vi "TSV_2_LV.vi"(8 "error in (no error)":errorcluster, 11 "tsv file path (dialog if empty)":path) -> (0 "error out":errorcluster, 2 "data":T2[](array[typedef]))   [LabVIEW 2019, in "VCL_2_DSC.lvclass"]
uses:
  VCL_2_DSC.lvclass
  typedefs/TSLtoLV-cluster.ctl
  <vilib>/Utility/file.llb/Read Delimited Spreadsheet (string).vi
  <userlib>/_OpenG.lib/array/array.llb/Index 1D Array Elements (String)__ogtk.vi
  <userlib>/_OpenG.lib/array/array.llb/Remove Duplicates from 1D Array (I32)__ogtk.vi
  <vilib>/Utility/file.llb/Read Delimited Spreadsheet (DBL).vi
  <userlib>/_OpenG.lib/array/array.llb/Delete Elements from 1D Array (DBL)__ogtk.vi
  <userlib>/_OpenG.lib/array/array.llb/Remove Duplicates from 1D Array (DBL)__ogtk.vi
  <userlib>/_OpenG.lib/array/array.llb/Index 1D Array Elements (Variant)__ogtk.vi
  <userlib>/_OpenG.lib/array/array.llb/Delete Elements from 1D Array (Variant)__ogtk.vi
  <userlib>/_OpenG.lib/array/array.llb/Filter 1D Array (DBL)__ogtk.vi
  <vilib>/addons/WireFlow/_WF_ProgressBar.llb/ProgressBar_WireFlow.lvclass
panel:
  in  "index 2":i32
  out "Waveform Graph":dbl[](graph)
  in  "index":i32
  out "XY Graph 2":T1(graph)
  out "XY Graph":T3(graph)
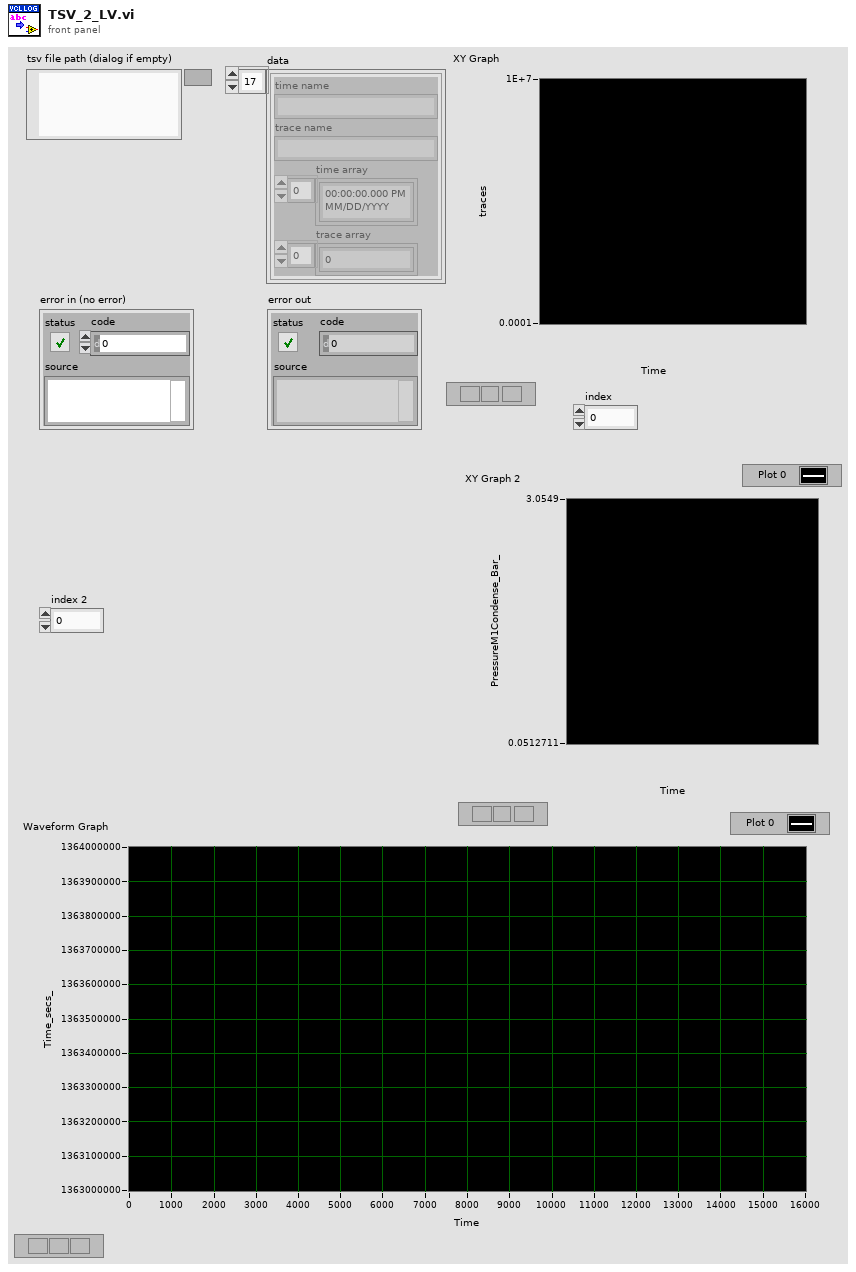
[diagram p1: front panel]
types:
  T1 = cluster{"time array":timestamp[], "trace array":dbl[]}
  T2 = typedef "VCL_2_DSC.lvclass/TSLtoLV-cluster.ctl" = cluster{"time name":string, "trace name":string, "time array":timestamp[], "trace array":dbl[]}
  T3 = cluster{"time array":timestamp[], "trace array":dbl[]}[]
  T4 = cluster{string, string, cluster{dbl[]}, cluster{dbl[]}}
  T5 = cluster{string, string, cluster{dbl[]}, cluster{dbl[]}}[]
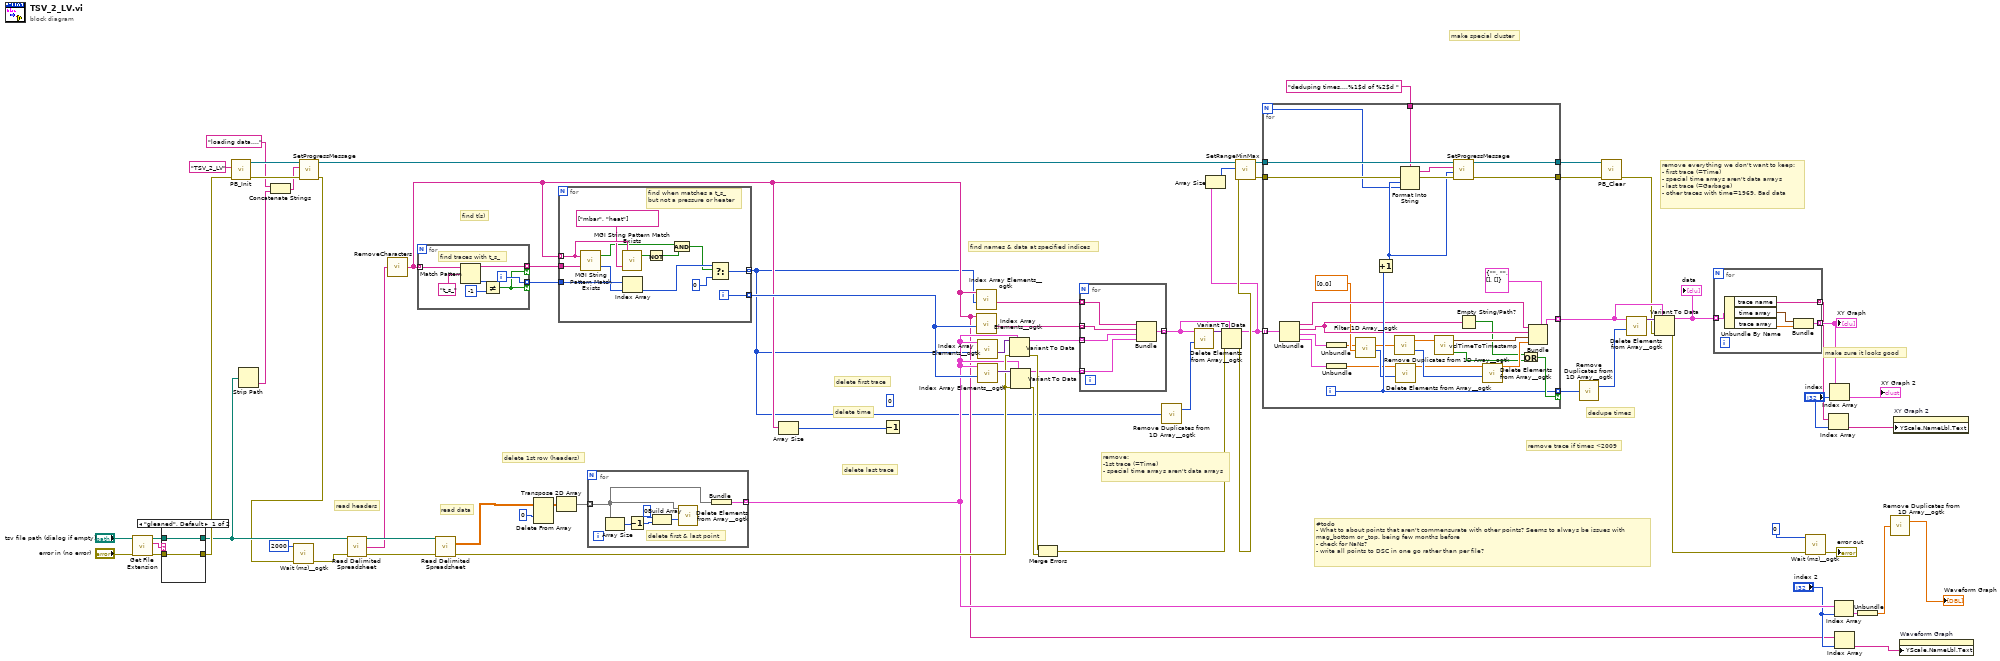
[diagram p0: block diagram]
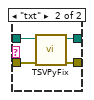
[diagram p2: hidden frame]
diagram:
  (unwired) 0 ("element")
  # "remove:\n-1st trace (=Time)\n- special time arrays aren't data arrays"
  # "#todo\n- What to about points that aren't commensurate with other points? Seems to always be issues with \nmag_bottom or _top. being few months before\n- check for NaNs?\n- write all points to DSC in one go rather than per file?"
  # "make sure it looks good"
  # "remove everything we don't want to keep:\n- first trace (=Time)\n- special time arrays aren't data arrays\n- last trace (=Garbage)\n- other traces with time=1969. Bad data"
  # "make special cluster"
  # "find names & data at specified indices"
  # "find t(s)"
  # "remove trace if times <2009"
  # "delete time"
  # "dedupe times"
  # "delete last trace"
  # "delete first trace"
  # "read data"
  # "delete 1st row (headers)"
  # "read headers"
  n1 = call <vilib>:"Get File Extension.vi"("error in (no error)"="error in (no error)", "file"="tsv file path (dialog if empty)") -> ("error out"=w4:errorcluster, "lowercase file extension"=w2:string, "dup file"=w1:path)  [unwired: 5 in, 2 out]
  n2 = case shown="\"gleaned\", Default" w2 {
    tunnel: [w72 w77] -> w16
    tunnel: [w73 w76] -> w15
    tunnel: w4 -> [w72 w75]
    tunnel: w1 -> [w73 w74]
    frame "gleaned", Default {
    }
    frame "txt" {
      n3 = call "TSVPyFix.vi"("error in (no error)"=w75, "Path to text file"=w74) -> ("error out"=w77:errorcluster, "Path to gleaned text file"=w76:path)  [unwired: 8 in]
    }
  }
  n4 = call <vilib>:"PB_Init.vi"("error in (no error)"=w16, "title (\"Progress\")"="TSV_2_LV" ("title (\"Progress\")")) -> ("error out"=w52:errorcluster, "WF-ProgressBar out"=w51:refnum<class "ProgressBar_WireFlow.lvclass">)  [unwired: 8 in]
  n5 = Strip Path(path=w15) -> (name=w14:string)  [unwired: 1 out]
  n6 = Concatenate Strings("loading data...." ("Message"), w14) -> (w42:string)
  n7 = call-dynamic "SetProgressMessage.vi"("error in (no error)"=w52, "Message"=w42, "WF-ProgressBar in"=w51) -> ("error out"=w11:errorcluster, "WF-ProgressBar out"=w50:refnum<class "ProgressBar_WireFlow.lvclass">)  [unwired: 6 in, 1 out]
  n8 = call <userlib>:"Wait (ms)__ogtk.vi"("error in (no error)"=w11, "milliseconds to wait"=u32 2000) -> ("error out"=w12:errorcluster)  [unwired: 8 in, 1 out]
  n9 = call-poly <vilib>:"Read Delimited Spreadsheet.vi"("file path (dialog if empty)"=w15, "error in (no error)"=w12) -> ("new file path (Not A Path if cancelled)"=w71:path, "first row"=w9:string[], "error out"=w69:errorcluster)  [unwired: 8 in, 3 out]
  n10 = call "RemoveCharacters.vi"("first row"=w9) -> ("Array"=w21:string[])
  n11 = for {
    tunnel: w21 -> [w83] mode=indexing
    tunnel: [w80] -> w48 mode=indexing if=w79
    tunnel: [w84] -> w47 mode=indexing if=w79
    i -> [w84]
    # "find traces with t_s_"
    n12 = Match Pattern(string=w83, regular expression="t_s_") -> (before substring=w80:string, offset past match=w81:i32)  [unwired: 1 in, 2 out]
    n13 = Not Equal?(x=w81, y=-1) -> (x != y?=w79:bool)
  }
  n14 = call-poly <vilib>:"Read Delimited Spreadsheet.vi"("file path (dialog if empty)"=w71, "error in (no error)"=w69) -> ("all rows"=w7:dbl[][], "error out"=w58:errorcluster)  [unwired: 8 in, 4 out]
  n15 = Delete From Array(array=w7, index (row)=0) -> (array with subset deleted=w64:dbl[][])  [unwired: 2 in, 1 out]
  n16 = Transpose 2D Array(2D array=w64) -> (transposed array=w68:dbl[][])
  n17 = for {
    tunnel: w48 -> [w97]
    tunnel: w47 -> [w93]
    tunnel: [w94] -> w8 mode=indexing
    tunnel: w21 -> [w90] mode=indexing
    tunnel: [w95] -> w41 mode=indexing
    i -> [w95]
    # "find when matches a t_s_\nbut not a pressure or heater"
    n18 = call <userlib>:"MGI String Pattern Match Exists.vi"("Patterns to Try"=w97, "String"=w90) -> ("Index of First Pattern Matched"=w91:i32, "Match Found"=w87:bool)
    n19 = call <userlib>:"MGI String Pattern Match Exists.vi"("Patterns to Try"=string[] ["mbar", "heat"], "String"=w90) -> ("Match Found"=w88:bool)  [unwired: 1 out]
    n20 = Index Array(array=w93, index=w91) -> (element=w92:i32)
    n21 = Not(x=w88) -> (.not. x?=w85:bool)
    n22 = And(x=w87, y=w85) -> (x .and. y?=w86:bool)
    n23 = Select(t=w92, s=w86, f=0) -> (s? t:f=w94:i32)
  }
  n24 = for {
    tunnel: w68 -> [w98] mode=indexing
    tunnel: [w103] -> w24 mode=indexing
    # "delete first & last point"
    n25 = Array Size(array=w98) -> (size(s)=w102:i32)
    n26 = Decrement(x=w102) -> (x-1=w101:i32)
    n27 = Build Array(0 ("element"), w101) -> (w99:i32[])
    n28 = call-poly <userlib>:"Delete Elements from Array__ogtk.vi"("indices"=w99, "array"=w98) -> ()  [unwired: 8 in, 2 out]
    n29 = Bundle(w98) -> (w103:cluster{dbl[]})  [unwired: 1 in]
  }
  n30 = Array Size(array=w21) -> (size(s)=w56:i32)
  n31 = Decrement(x=w56) -> ()  [unwired: 1 out]
  n32 = call-poly <userlib>:"Index Array Elements__ogtk.vi"("indices"=w8, "array"=w21) -> ("elements"=w40:string[])  [unwired: 9 in]
  n33 = call-poly <userlib>:"Index Array Elements__ogtk.vi"("indices"=w41, "array"=w21) -> ("elements"=w39:string[])  [unwired: 9 in]
  n34 = call-poly <userlib>:"Index Array Elements__ogtk.vi"("indices"=w8, "array"=w24) -> ("elements"=w63:variant[])  [unwired: 9 in]
  n35 = call-poly <userlib>:"Index Array Elements__ogtk.vi"("indices"=w41, "array"=w24) -> ("elements"=w62:variant[])  [unwired: 9 in]
  n36 = Variant To Data(error in=w58, type=w24, Variant=w63) -> (data=w38:cluster{dbl[]}[], error out=w60:errorcluster)
  n37 = Variant To Data(error in=w58, type=w24, Variant=w62) -> (data=w37:cluster{dbl[]}[], error out=w59:errorcluster)
  n38 = Merge Errors(w60, w59) -> (w34:errorcluster)
  n39 = for {
    tunnel: w40 -> [w108] mode=indexing
    tunnel: w39 -> [w107] mode=indexing
    tunnel: w38 -> [w106] mode=indexing
    tunnel: w37 -> [w105] mode=indexing
    tunnel: [w104] -> w35 mode=indexing
    n40 = Bundle(w108, w107, w106, w105) -> (w104:T4)  [unwired: 1 in]
  }
  n41 = call-poly <userlib>:"Remove Duplicates from 1D Array__ogtk.vi"("Input Array"=w8) -> ("Output Array"=w6:i32[])  [unwired: 1 out]
  n42 = call-poly <userlib>:"Delete Elements from Array__ogtk.vi"("indices"=w6, "array"=w35) -> ("array w/ subset deleted"=w36:variant[])  [unwired: 8 in, 1 out]
  n43 = Variant To Data(error in=w34, type=w35, Variant=w36) -> (data=w32:T5, error out=w33:errorcluster)
  n44 = Array Size(array=w32) -> (size(s)=w55:i32)
  n45 = call-dynamic "SetRangeMinMax.vi"("error in (no error)"=w33, "Max (1)"=w55, "WF-ProgressBar in"=w50) -> ("error out"=w46:errorcluster, "WF-ProgressBar out"=w45:refnum<class "ProgressBar_WireFlow.lvclass">)  [unwired: 7 in]
  n46 = for {
    N -> [w117]
    tunnel: [w138] -> w65 mode=indexing
    tunnel: [w130] -> w31 mode=indexing if=w132
    tunnel: w46 -> [w131]
    tunnel: w45 -> [w127]
    tunnel: "deduping times....%1$d of %2$d " ("format string") -> [w124]
    tunnel: [w128] -> w43
    tunnel: [w129] -> w44
    tunnel: w32 -> [w123] mode=indexing
    i -> [w130]
    n47 = Unbundle(w123) -> (w122:string, w121:string, w120:cluster{dbl[]}, w119:cluster{dbl[]})
    n48 = Unbundle(w120) -> (w113:dbl[])
    n49 = Unbundle(w119) -> (w111:dbl[])
    n50 = call-poly <userlib>:"Filter 1D Array__ogtk.vi"("items to filter"=dbl[] [0.0], "array"=w113) -> ("filtered item indices"=w114:i32[], "filtered array"=w112:dbl[])  [unwired: 4 in]
    n51 = Increment(x=w130) -> (x+1=w118:i32)
    n52 = call-poly <userlib>:"Remove Duplicates from 1D Array__ogtk.vi"("Input Array"=w112) -> ("Output Array"=w135:dbl[], "indices of removed elements"=w134:i32[])
    n53 = call-poly <userlib>:"Delete Elements from Array__ogtk.vi"("indices"=w114, "array"=w111) -> ("array w/ subset deleted"=w110:dbl[])  [unwired: 8 in, 1 out]
    n54 = Format Into String(format string=w124, error in=w131, w118, w117) -> (resulting string=w125:string, error out=w126:errorcluster)  [unwired: 1 in]
    n55 = call "vclTimeToTimestamp.vi"("all rows"=w135) -> ("before 2009?"=w116:bool, "Array"=w133:timestamp[])  [unwired: 1 in]
    n56 = call-dynamic "SetProgressMessage.vi"("error in (no error)"=w126, "Progress value (NaN no update)"=w118, "Message"=w125, "WF-ProgressBar in"=w127) -> ("error out"=w129:errorcluster, "WF-ProgressBar out"=w128:refnum<class "ProgressBar_WireFlow.lvclass">)  [unwired: 5 in, 1 out]
    n57 = Empty String/Path?(string/path=w121) -> (empty?=w109:bool)
    n58 = call-poly <userlib>:"Delete Elements from Array__ogtk.vi"("indices"=w134, "array"=w110) -> ("array w/ subset deleted"=w136:dbl[])  [unwired: 8 in, 1 out]
    n59 = Or(x=w109, y=w116) -> (x .or. y?=w132:bool)
    n60 = Bundle(cluster=T2 {"time name"="", "trace name"="", "time array"=[], "trace array"=[]}, "time name"=w122, "trace name"=w121, "time array"=w133, "trace array"=w136) -> (w138:T2)
  }
  n61 = call-poly <userlib>:"Remove Duplicates from 1D Array__ogtk.vi"("Input Array"=w31) -> ("Output Array"=w30:i32[])  [unwired: 1 out]
  n62 = call-dynamic "PB_Clear.vi"("error in (no error)"=w44, "WF-ProgressBar in"=w43) -> ("error out"=w53:errorcluster)  [unwired: 8 in, 1 out]
  n63 = call-poly <userlib>:"Delete Elements from Array__ogtk.vi"("indices"=w30, "array"=w65) -> ("array w/ subset deleted"=w66:variant[])  [unwired: 8 in, 1 out]
  n64 = Variant To Data(error in=w53, type=w65, Variant=w66) -> (data=w29:T2[], error out=w57:errorcluster)
  "data" <- w29
  n65 = for {
    tunnel: w29 -> [w142] mode=indexing
    tunnel: [w141] -> w28 mode=indexing
    tunnel: [w139] -> w27 mode=indexing
    n66 = Unbundle By Name(w142) -> ("trace name"=w139:string, "time array"=w140:timestamp[], "trace array"=w143:dbl[])
    n67 = Bundle("time array"=w140, "trace array"=w143) -> (w141:T1)  [unwired: 1 in]
  }
  "XY Graph" <- w28
  n68 = call <userlib>:"Wait (ms)__ogtk.vi"("error in (no error)"=w57, "milliseconds to wait"=u32 0) -> ("error out"=→"error out":errorcluster)  [unwired: 8 in, 1 out]
  n69 = Index Array(array=w27, index="index") -> (element=w25:string)
  n70 = Index Array(array=w28, index="index") -> (element=→"XY Graph 2":T1)
  n71 = Index Array(array=w24, index="index 2") -> (element=w23:cluster{dbl[]})
  n72 = Index Array(array=w21, index="index 2") -> (element=w20:string)
  n73 = Unbundle(w23) -> (w18:dbl[])
  n74 = call-poly <userlib>:"Remove Duplicates from 1D Array__ogtk.vi"("Input Array"=w18) -> ("Output Array"=→"Waveform Graph":dbl[])  [unwired: 1 out]
  n75 = property on="XY Graph 2" class="XYGraph (strict)"("YScale.NameLbl.Text"=w25) -> ()  [unwired: 2 in, 2 out]
  n76 = property on="Waveform Graph" class="WFGraph (strict)"("YScale.NameLbl.Text"=w20) -> ()  [unwired: 2 in, 2 out]
